vi "text adding (Biswajit).vi"(1 "string":string, 2 "number":dbl) -> (0 "String":string)   [LabVIEW 2025, in "Cryo.lvlib"]
uses:
  Cryo.lvlib
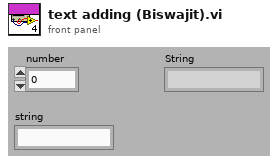
[diagram p1: front panel]
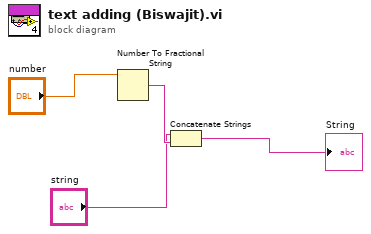
[diagram p0: block diagram]
diagram:
  n1 = Number To Fractional String(number="number") -> (F-format string=w2:string)  [unwired: 3 out]
  n2 = Concatenate Strings("string", w2) -> (→"String":string)
